vi "Get-New-iteration.vi"(8 "error in (no error)":errorcluster, 11 "UI ref. in":refnum<data-value>) -> (0 "error out":errorcluster, 1 "New iteration":bool, 3 "UI ref.":refnum<data-value>)   [LabVIEW 2013, in "CameraVision.lvlib" / "CV-UI.lvclass"]
uses:
  CV-UI.lvclass
  CV-UI.lvclass/CV-UI.ctl
  Notifier-with-memory-boolean.vi
  Read IterationTrigger.vi
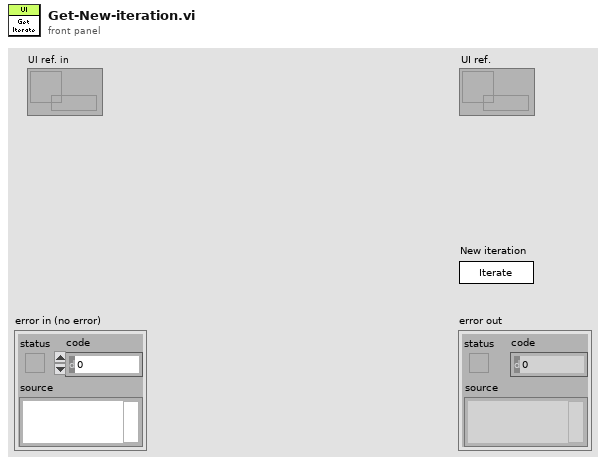
[diagram p1: front panel]
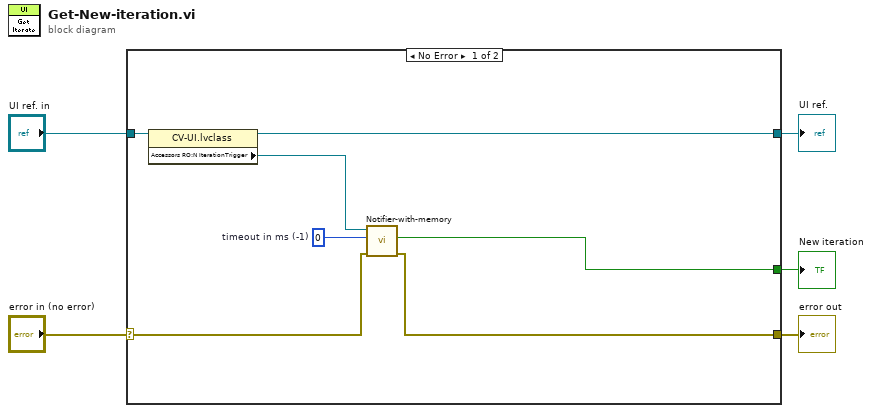
[diagram p0: block diagram]
diagram:
  n1 = case shown="No Error" "error in (no error)" {
    selector: "error in (no error)" -> [w6 w14]
    tunnel: [w9 w14] -> w4
    tunnel: "UI ref. in" -> [w12 w13]
    tunnel: [w11 w13] -> w2
    tunnel: [w10 _] -> w1
    frame No Error {
      w8 = 0  # timeout in ms (-1)
      n2 = property class="CV-UI.lvclass"(reference=w12) -> (reference out=w11:refnum<data-value>, "Accessors RO:N IterationTrigger"=w7:refnum<notifier>)  [unwired: 1 in, 1 out]
      n3 = call-poly "Notifier-with-memory.vi"("error in"=w6, "Timeout [ms]"=w8, "Notifier in"=w7) -> ("error IO"=w9:errorcluster, "Notification"=w10:bool)  [unwired: 7 in]
    }
    frame Error {
    }
  }
  "error out" <- w4
  "UI ref." <- w2
  "New iteration" <- w1
